vi "多参数电源命令.vi"(10 "通电/断电":bool, 11 "队列":refnum<queue>) -> (3 "队列输出":refnum<queue>)   [LabVIEW 2016, in "环境动力监测库.lvlib" / "G电源管理库.lvlib"]
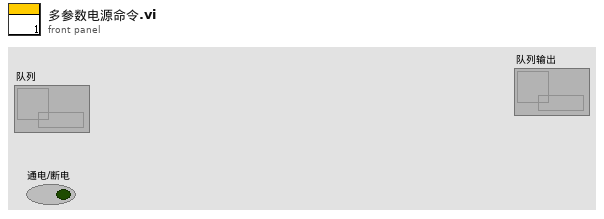
[diagram p1: front panel]
types:
  T1 = cluster{"命令":string, "data":cluster{"starting address":u16, "coil values":bool[]}}
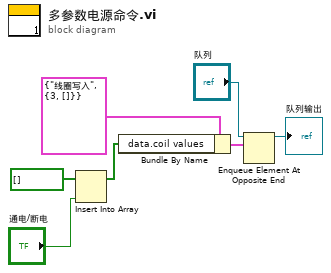
[diagram p0: block diagram]
diagram:
  n1 = Insert Into Array(array=bool[] [] ("data.coil values"), new element="通电/断电") -> (w2:bool[])  [unwired: 1 in]
  n2 = Bundle By Name(cluster=T1 {"命令"="线圈写入", "data"={"starting address"=3, "coil values"=[]}} ("元素"), "data.coil values"=w2) -> (w6:T1)
  n3 = Enqueue Element At Opposite End(queue="队列", element=w6) -> (queue out=→"队列输出":refnum<queue>)  [unwired: 2 in, 2 out]
